vi "timer.vi"() -> ()   [LabVIEW 2019]
panel:
  out "stop":bool
  out "elapsed time":dbl
  in  "tijdsinterval":dbl
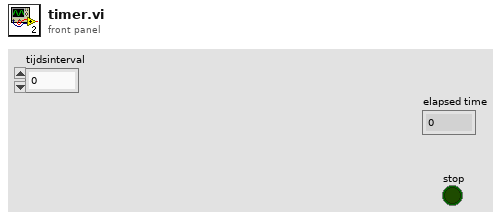
[diagram p1: front panel]
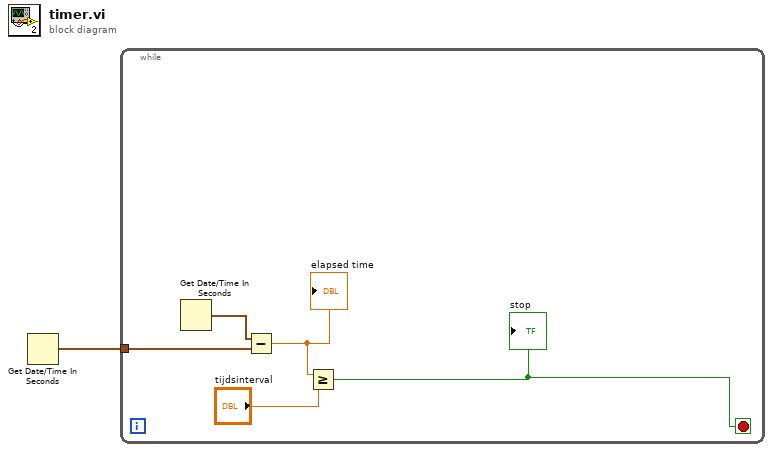
[diagram p0: block diagram]
diagram:
  n1 = Get Date/Time In Seconds() -> (seconds since 1Jan1904=w1:timestamp)
  n2 = while {
    tunnel: w1 -> [w5]
    stop <- w2 stop-if-true
    n3 = Get Date/Time In Seconds() -> (seconds since 1Jan1904=w6:timestamp)
    n4 = Subtract(x=w6, y=w5) -> (x-y=w3:dbl)
    "elapsed time" <- w3
    n5 = Greater Or Equal?(x=w3, y="tijdsinterval") -> (x >= y?=w2:bool)
    "stop" <- w2
  }
